vi "rethinkdb_json_db.vi"(7 "action":enum8{"get", "push", "pop"}(ring), 8 "error in (no error)":errorcluster, 10 "cluster in":variant, 11 "id in":u64) -> (0 "error out":errorcluster, 1 "exists?":bool, 2 "cluster out":variant, 3 "id out":u64)   [LabVIEW 2017]
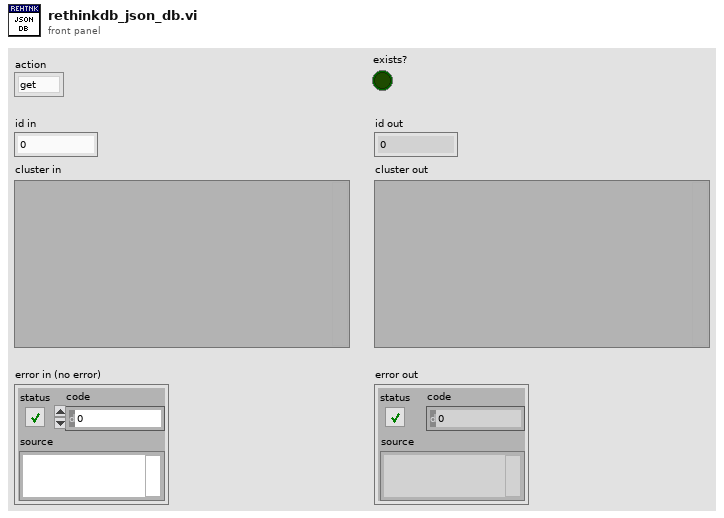
[diagram p1: front panel]
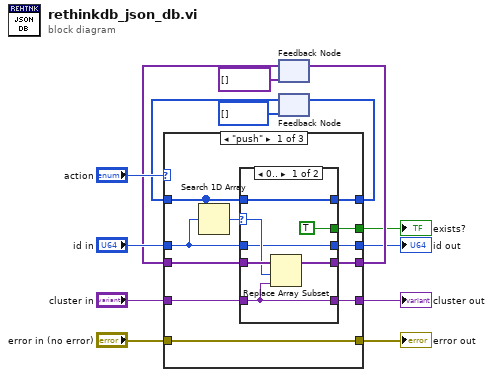
[diagram p0: block diagram]
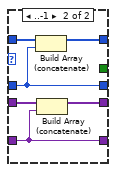
[diagram p2: hidden frame]
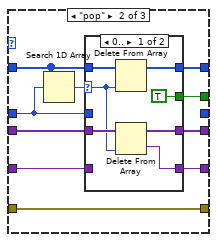
[diagram p3: hidden frame]
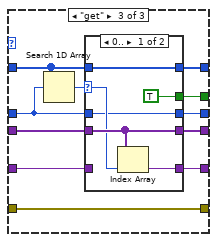
[diagram p5: hidden frame]
diagram:
  n1 = feedback #1(variant[] []) -> (w8:variant[])
  n2 = feedback #2(u64[] []) -> (w11:u64[])
  n3 = case shown="\"push\"" "action" {
    tunnel: w11 -> [w24 w47 w68]
    tunnel: "id in" -> [w20 w43 w64]
    tunnel: [w25 w48 w69] -> w9
    tunnel: w8 -> [w23 w46 w67]
    tunnel: [w22 w45 w66] -> w7
    tunnel: "cluster in" -> [w18 w41 w62]
    tunnel: [w19 w42 w63] -> w5
    tunnel: "error in (no error)" -> [w19 w42 w63]
    tunnel: [w16 _ w60] -> w3
    tunnel: [w17 w40 w61] -> w2
    tunnel: [w15 w39 w59] -> w1
    frame "push" {
      n4 = Search 1D Array(1D array=w24, element=w20) -> (index of element=w21:i32)  [unwired: 1 in]
      n5 = case shown="0.." w21 {
        selector: w21 -> [w30 _]
        tunnel: [w32 w38] -> w25
        tunnel: w24 -> [w32 w37]
        tunnel: w23 -> [w31 w36]
        tunnel: [w29 w35] -> w22
        tunnel: w20 -> [w27 w33]
        tunnel: w18 -> [w28 w34]
        tunnel: [w28 w34] -> w17
        tunnel: [w27 w33] -> w16
        tunnel: [TRUE _] -> w15
        frame 0.. {
          n6 = Replace Array Subset(array=w31, new element=w28, index=w30) -> (w29:variant[])
        }
        frame ..-1 {
          n7 = Build Array (concatenate)(w37, w33) -> (w38:u64[])
          n8 = Build Array (concatenate)(w36, w34) -> (w35:variant[])
        }
      }
    }
    frame "pop" {
      n9 = Search 1D Array(1D array=w47, element=w43) -> (index of element=w44:i32)  [unwired: 1 in]
      n10 = case shown="0.." w44 {
        selector: w44 -> [w51 _]
        tunnel: [w52 w58] -> w48
        tunnel: w47 -> [w53 w58]
        tunnel: w46 -> [w55 w57]
        tunnel: [w54 w57] -> w45
        tunnel: w43 -> [_ _]
        tunnel: w41 -> [_ w56]
        tunnel: [w50 w56] -> w40
        tunnel: [TRUE _] -> w39
        frame 0.. {
          n11 = Delete From Array(array=w53, index=w51) -> (array with subset deleted=w52:u64[])  [unwired: 1 in, 1 out]
          n12 = Delete From Array(array=w55, index=w51) -> (deleted portion=w50:variant, array with subset deleted=w54:variant[])  [unwired: 1 in]
        }
        frame ..-1 {
        }
      }
    }
    frame "get" {
      n13 = Search 1D Array(1D array=w68, element=w64) -> (index of element=w65:i32)  [unwired: 1 in]
      n14 = case shown="0.." w65 {
        selector: w65 -> [w73 _]
        tunnel: [w75 w79] -> w69
        tunnel: w68 -> [w75 w79]
        tunnel: w67 -> [w74 w78]
        tunnel: [w74 w78] -> w66
        tunnel: w64 -> [w71 w76]
        tunnel: w62 -> [_ w77]
        tunnel: [w72 w77] -> w61
        tunnel: [w71 w76] -> w60
        tunnel: [TRUE _] -> w59
        frame 0.. {
          n15 = Index Array(array=w74, index=w73) -> (element=w72:variant)
        }
        frame ..-1 {
        }
      }
    }
  }
  "error out" <- w5
  "id out" <- w3
  "cluster out" <- w2
  "exists?" <- w1
  n16 = feedback-in #1(w7) -> ()
  n17 = feedback-in #2(w9) -> ()
